vi "GDSLvIcon_FloodFill.vi"(6 "4 (T) or 8 (F)":bool, 7 "NewColor":u8, 8 "error in (no error)":errorcluster, 9 "StartPositions":cluster{"x":i32, "y":i32}[](array[cluster]), 11 "IconIn":u8[][](array[numeric])=[[9, 9, 9, 0, 0, 0, 0, 0, 0, 0, 0], [9, 9, 9, 9, 0, 0, 0, 0, 0, 0, 0], [0, 9, 9, 9, 0, 0, 0, 0, 0, 0, 0], [0, 9, 9, 9, 9, 9, 0, 0, 0, 0, 0], [0, 0, 0, 0, 9, 9, 9, 0, 0, 0, 0], [0, 0, 0, 0, 0, 9, 9, 0, 0, 0, 0], [0, 0, 0, 0, 0, 0, 0, 0, 0, 0, 0], [0, 0, 0, 0, 0, 0, 0, 0, 0, 0, 0], [0, 0, 0, 0, 0, 0, 0, 0, 0, 0, 0]] format="%x") -> (0 "error out":errorcluster, 2 "PointsFilled":cluster{"y":i32, "x":i32}[](array[cluster]), 3 "IconOut":u8[][](array[numeric])=[[9, 9, 9, 0, 0, 0, 0, 0, 0, 0, 0], [9, 9, 9, 9, 0, 0, 0, 0, 0, 0, 0], [0, 9, 9, 9, 0, 0, 0, 0, 0, 0, 0], [0, 9, 9, 9, 9, 9, 0, 0, 0, 0, 0], [0, 0, 0, 0, 9, 9, 9, 0, 0, 0, 0], [0, 0, 0, 0, 0, 9, 9, 0, 0, 0, 0], [0, 0, 0, 0, 0, 0, 0, 0, 0, 0, 0], [0, 0, 0, 0, 0, 0, 0, 0, 0, 0, 0], [0, 0, 0, 0, 0, 0, 0, 0, 0, 0, 0]] format="%.0x")   [LabVIEW 2020]
doc: "Wiebe Walstra.\nCarya Automatisering\nwww.carya.nl"
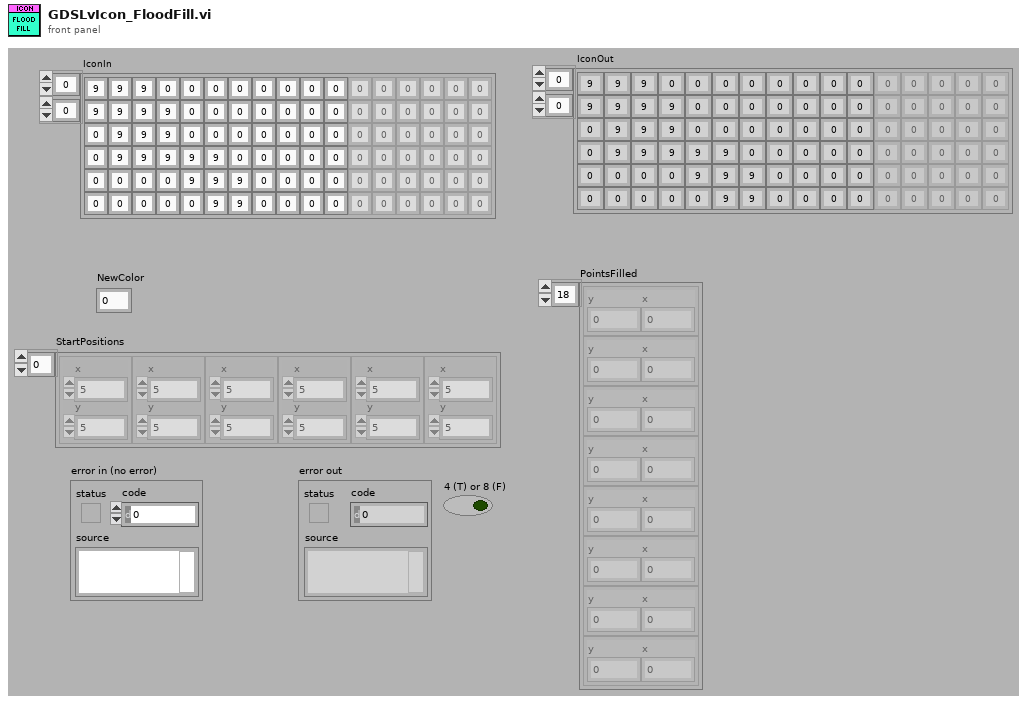
[diagram p1: front panel]
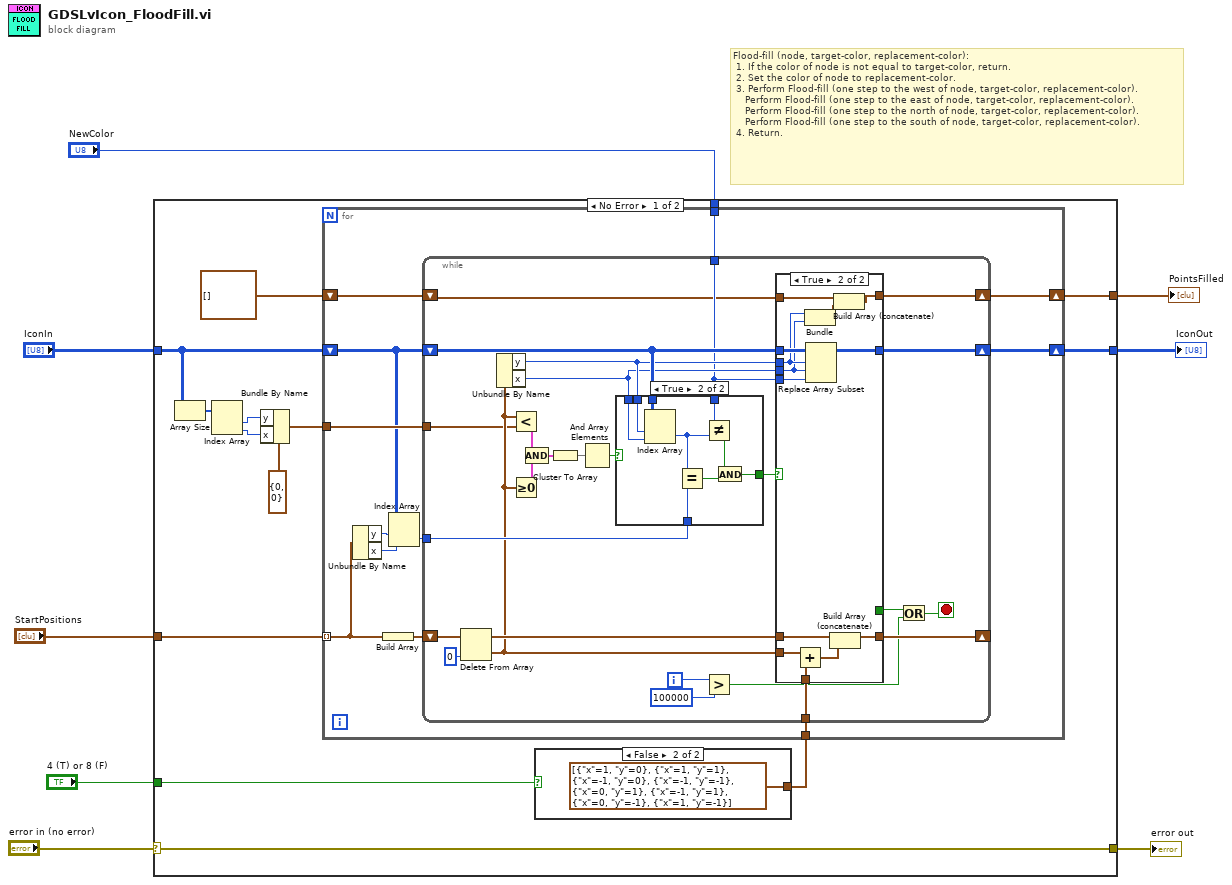
[diagram p0: block diagram]
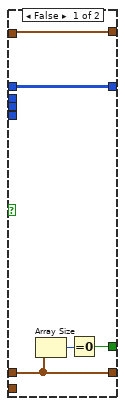
[diagram p3: hidden frame]
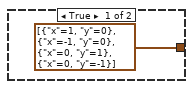
[diagram p4: hidden frame]
diagram:
  # "Flood-fill (node, target-color, replacement-color):\n 1. If the color of node is not equal to target-color, return.\n 2. Set the color of node to replacement-color.\n 3. Perform Flood-fill (one step to the west of node, target-color, replacement-color).\n    Perform Flood-fill (one step to the east of node, target-color, replacement-color).\n    Perform Flood-fill (one step to the north of node, target-color, replacement-color).\n    Perform Flood-fill (one step to the south of node, target-color, replacement-color).\n 4. Return."
  n1 = case shown="No Error" "error in (no error)" {
    selector: "error in (no error)" -> [w16 w91]
    tunnel: [w16 w91] -> w7
    tunnel: "StartPositions" -> [w15 _]
    tunnel: "IconIn" -> [w14 _]
    tunnel: [w13 _] -> w4
    tunnel: [w12 _] -> w3
    tunnel: "NewColor" -> [w11 _]
    tunnel: "4 (T) or 8 (F)" -> [w10 _]
    frame No Error {
      n2 = Array Size(array=w14) -> (size(s)=w22:i32[])
      n3 = Index Array(array=w22) -> (element #1=w21:i32, element #2=w20:i32)  [unwired: 2 in]
      n4 = Bundle By Name(cluster=cluster{"x":i32, "y":i32} {"x"=0, "y"=0} ("input cluster"), "y"=w21, "x"=w20) -> (w19:cluster{"x":i32, "y":i32})
      n5 = case shown="False" w10 {
        tunnel: [cluster{"x":i32, "y":i32}[] [{"x"=1, "y"=0}, {"x"=-1, "y"=0}, {"x"=0, "y"=1}, {"x"=0, "y"=-1}] cluster{"x":i32, "y":i32}[] [{"x"=1, "y"=0}, {"x"=1, "y"=1}, {"x"=-1, "y"=0}, {"x"=-1, "y"=-1}, {"x"=0, "y"=1}, {"x"=-1, "y"=1}, {"x"=0, "y"=-1}, {"x"=1, "y"=-1}]] -> w18
        frame True {
        }
        frame False {
        }
      }
      n6 = for {
        tunnel: w19 -> [w30]
        tunnel: w18 -> [w29]
        tunnel: w15 -> [w27] mode=indexing
        tunnel: w11 -> [w23]
        shift-right: [w24] -> w12
        shift-left: w14 -> [w26]
        shift-right: [w25] -> w13
        shift-left: cluster{"y":i32, "x":i32}[] [] -> [w28]
        n7 = Unbundle By Name(w27) -> ("y"=w33:i32, "x"=w32:i32)
        n8 = Build Array(w27) -> (w34:cluster{"x":i32, "y":i32}[])
        n9 = Index Array(array=w26, index (row)=w33, index (col)=w32) -> (element=w31:u8)
        n10 = while {
          shift-right: [w60] -> w24
          shift-left: w26 -> [w58]
          shift-right: [w57] -> _
          shift-left: w34 -> [w56]
          tunnel: w31 -> [w53]
          tunnel: w30 -> [w49]
          tunnel: w23 -> [w43]
          tunnel: w29 -> [w42]
          shift-right: [w40] -> w25
          shift-left: w28 -> [w41]
          i -> [w39]
          stop <- w35 stop-if-true
          n11 = Delete From Array(array=w56, index=0) -> (deleted portion=w50:cluster{"x":i32, "y":i32}, array with subset deleted=w55:cluster{"x":i32, "y":i32}[])  [unwired: 1 in]
          n12 = Unbundle By Name(w50) -> ("y"=w45:i32, "x"=w44:i32)
          n13 = Less?(x=w50, y=w49) -> (x < y?=w52:cluster{"x":bool, "y":bool})
          n14 = Greater Or Equal To 0?(x=w50) -> (x >= 0?=w51:cluster{"x":bool, "y":bool})
          n15 = Compound Arithmetic op=AND(w52, w51) -> (w48:cluster{"x":bool, "y":bool})
          n16 = Cluster To Array(cluster=w48) -> (array=w47:bool[])
          n17 = And Array Elements(Boolean array=w47) -> (logical AND=w46:bool)
          n18 = case shown="True" w46 {
            selector: w46 -> [w61 _]
            tunnel: w58 -> [_ w70]
            tunnel: [w61 w68] -> w59
            tunnel: w53 -> [_ w69]
            tunnel: w43 -> [_ w64]
            tunnel: w45 -> [_ w67]
            tunnel: w44 -> [_ w66]
            frame False {
            }
            frame True {
              n19 = Index Array(array=w70, index (row)=w67, index (col)=w66) -> (element=w65:u8)
              n20 = Equal?(x=w65, y=w69) -> (x = y?=w63:bool)
              n21 = Not Equal?(x=w64, y=w65) -> (x != y?=w62:bool)
              n22 = And(x=w62, y=w63) -> (x .and. y?=w68:bool)
            }
          }
          n23 = Greater?(x=w39, y=100000) -> (0:w36:bool)
          n24 = case shown="True" w59 {
            tunnel: w58 -> [w75 w88]
            tunnel: [w75 w87] -> w60
            tunnel: w43 -> [_ w86]
            tunnel: w44 -> [_ w78]
            tunnel: w45 -> [_ w79]
            tunnel: w50 -> [_ w83]
            tunnel: w55 -> [w73 w85]
            tunnel: [w73 w84] -> w57
            tunnel: w42 -> [_ w82]
            tunnel: [w72 _] -> w37
            tunnel: w41 -> [w71 w80]
            tunnel: [w71 w76] -> w40
            frame False {
              n25 = Array Size(array=w73) -> (size(s)=w74:i32)
              n26 = Equal To 0?(x=w74) -> (x = 0?=w72:bool)
            }
            frame True {
              n27 = Add(x=w83, y=w82) -> (x+y=w81:cluster{"x":i32, "y":i32}[])
              n28 = Bundle("y"=w79, "x"=w78) -> (w77:cluster{"y":i32, "x":i32})  [unwired: 1 in]
              n29 = Replace Array Subset(array=w88, new element=w86, index (row)=w79, index (col)=w78) -> (w87:u8[][])
              n30 = Build Array (concatenate)(w85, w81) -> (w84:cluster{"x":i32, "y":i32}[])
              n31 = Build Array (concatenate)(w80, w77) -> (w76:cluster{"y":i32, "x":i32}[])
            }
          }
          n32 = Or(x=w37, y=w36) -> (x .or. y?=w35:bool)
        }
      }
    }
    frame Error {
    }
  }
  "error out" <- w7
  "IconOut" <- w3
  "PointsFilled" <- w4
